vi "Random Second.vi"(10 "Min Second":i32, 11 "Max Second":i32) -> (3 "Random Second":dbl format="%.2f")   [LabVIEW 2020]
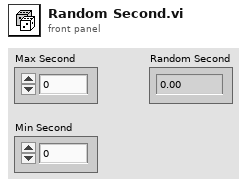
[diagram p1: front panel]
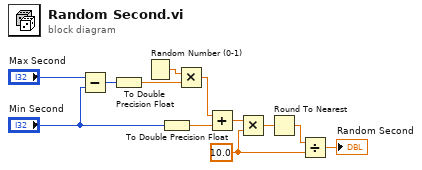
[diagram p0: block diagram]
diagram:
  w1 = 10.0 ("x")
  n1 = Subtract(x="Max Second", y="Min Second") -> (x-y=w12:i32)
  n2 = To Double Precision Float(number=w12) -> (double precision float=w8:dbl)
  n3 = Random Number (0-1)() -> (number: 0 to 1=w7:dbl)
  n4 = To Double Precision Float(number="Min Second") -> (double precision float=w9:dbl)
  n5 = Multiply(x=w7, y=w8) -> (x*y=w6:dbl)
  n6 = Add(x=w6, y=w9) -> (x+y=w5:dbl)
  n7 = Multiply(x=w5, y=w1) -> (x*y=w4:dbl)
  n8 = Round To Nearest(number=w4) -> (nearest integer value=w3:dbl)
  n9 = Divide(x=w3, y=w1) -> (x/y=→"Random Second":dbl)
